vi "Update Brownout Status.vi"(6 "VBus":dbl[unit], 8 "Timestep":dbl[unit], 9 "Battery Voltage":dbl[unit], 10 "Brownout in":cluster{bool, u32}) -> (2 "Brownout status":cluster{bool, u32}, 3 "Motor Voltage":dbl[unit])   [LabVIEW 2019]
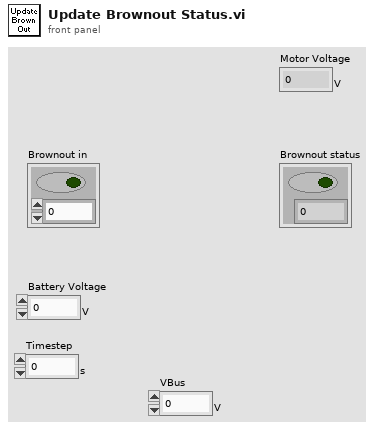
[diagram p1: front panel]
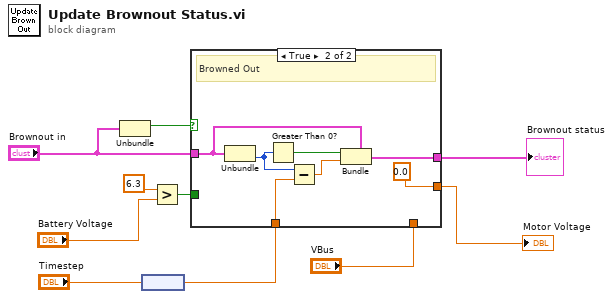
[diagram p0: block diagram]
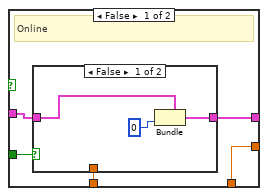
[diagram p2: hidden frame]
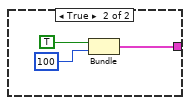
[diagram p3: hidden frame]
diagram:
  n1 = Unbundle("Brownout in") -> (w3:bool)  [unwired: 1 out]
  n2 = node("Timestep") -> (w1:dbl)
  n3 = Greater?(x=dbl[unit] 6.3 ("y"), y="Battery Voltage") -> (0:w7:bool)
  n4 = case shown="True" w3 {
    tunnel: [w14 w27] -> w8
    tunnel: "Brownout in" -> [w13 w26]
    tunnel: w7 -> [w15 _]
    tunnel: "VBus" -> [w12 _]
    tunnel: [w12 dbl[unit] 0.0 ("When Above")] -> w10
    tunnel: w1 -> [w11 w22]
    frame False {
      # "Online"
      n5 = case shown="False" w15 {
        tunnel: [w18 w20] -> w14
        tunnel: w13 -> [w16 _]
        tunnel: w11 -> [_ _]
        frame False {
          n6 = Bundle(cluster=w16, 0) -> (w18:cluster{bool, u32})  [unwired: 1 in]
        }
        frame True {
          n7 = Bundle(TRUE, 100) -> (w20:cluster{bool, i32})  [unwired: 1 in]
        }
      }
    }
    frame True {
      # "Browned Out"
      n8 = Unbundle(w26) -> (w24:u32)  [unwired: 1 out]
      n9 = Greater Than 0?(x=w24) -> (x > 0?=w28:bool)
      n10 = Subtract(x=w24, y=w22) -> (x-y=w23:dbl)
      n11 = Bundle(cluster=w26, w28, w23) -> (w27:cluster{bool, u32})
    }
  }
  "Motor Voltage" <- w10
  "Brownout status" <- w8
